vi "train_auto (deprecated).vi"() -> ()   [LabVIEW 2024]
uses:
  <vilib>/userDefined/High Color/IMAQdx.ctl
  <vilib>/vision/driver/NI_Vision_Acquisition_Software.lvlib
  <vilib>/vision/NI_Vision_Development_Module.lvlib
panel:
  in  "Set":enum16{"Train", "Test"}(ring)
  in  "Time Target (s)":dbl=0.4 min=0.1 max=20.0 step=0.1
  in  "Reset Set":bool
  in  "Update ROI":bool
  out "Original Image":T1(plugin-control)
  out "Time":dbl caption="Elapsed Time (s)"
  out "Toma":i32
  out "ROI":T1(plugin-control)
  in  "Save":bool
  in  "No. de Carta":i32
  in  "Path":string[](array[string])=["C:\\Users\\cesar\\OneDrive\\Universidad\\8vo Semestre\\Instrumentación Virtual 2\\Final\\cards\\train\\", "C:\\Users\\cesar\\OneDrive\\Universidad\\8vo Semestre\\Instrumentación Virtual 2\\Final\\cards\\test\\"]
  in  "Y":i32=150
  in  "X":i32=132
  out "Scaled ROI":T1(plugin-control)
  in  "ROI":T2={"Global Rectangle"=[408, 127, 510, 269], "Contours"=[{"Contour Type"=0, "ROI Type"=3, "Points"=[405, 125, 515, 272]}]}
  in  "Session In":T3="cam2"
  in  "Stop":bool
  # "Scale"
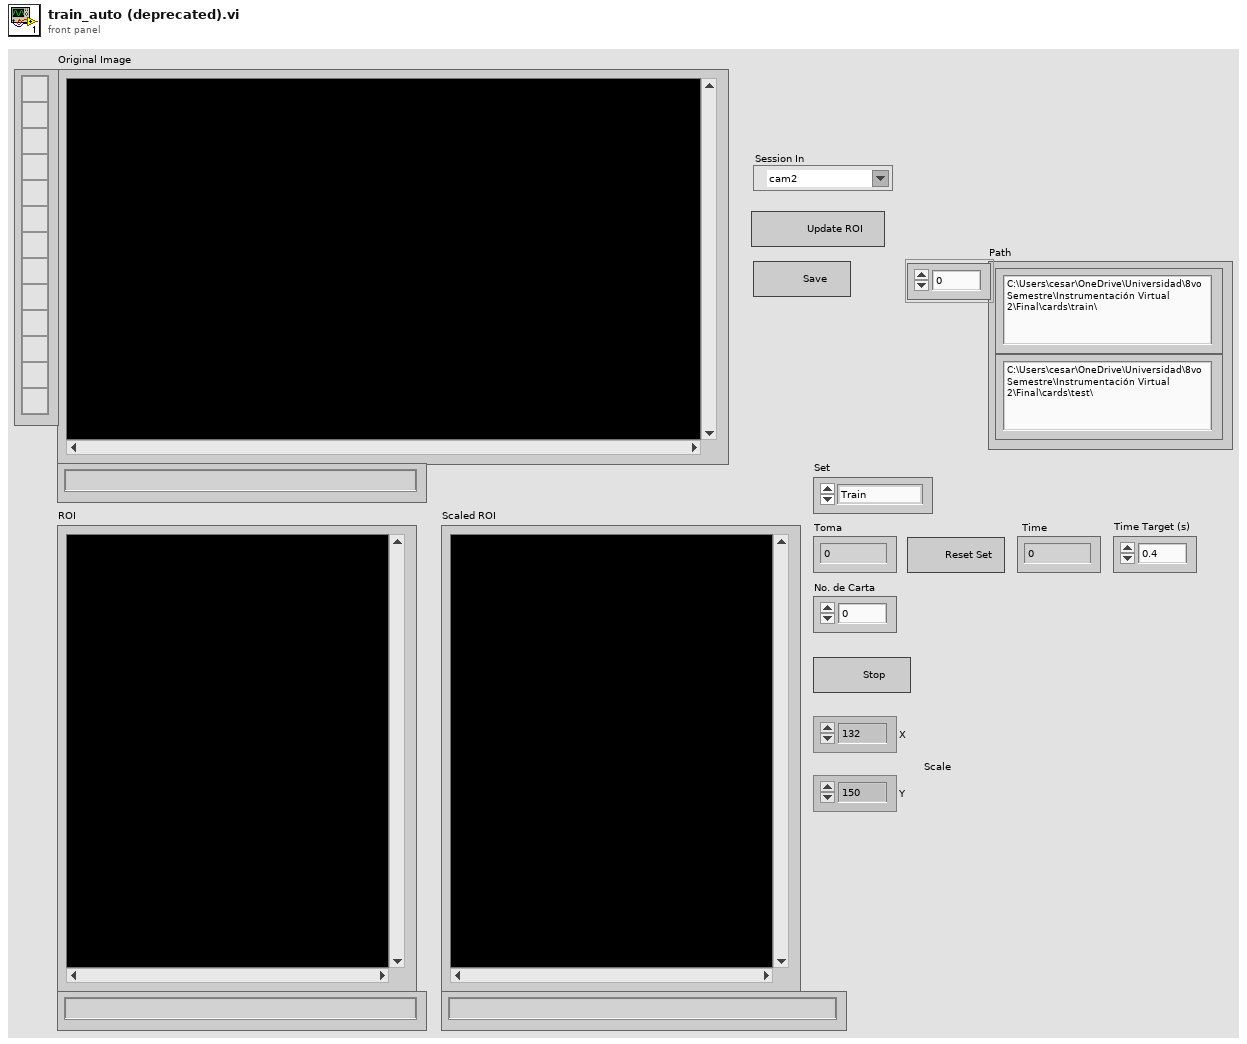
[diagram p1: front panel]
types:
  T1 = typedef "IMAQ Image.ctl" = refnum<image>
  T2 = cluster{"Global Rectangle":i32[], "Contours":cluster{"Contour Type":u32, "ROI Type":u32, "Points":i32[]}[]}
  T3 = typedef "IMAQdx.ctl" = refnum<k21>
  T4 = cluster{"Contour Type":u32, "ROI Type":u32, "Points":i32[]}[]
  T5 = cluster{"Contour Type":u32, "ROI Type":u32, "Points":i32[]}
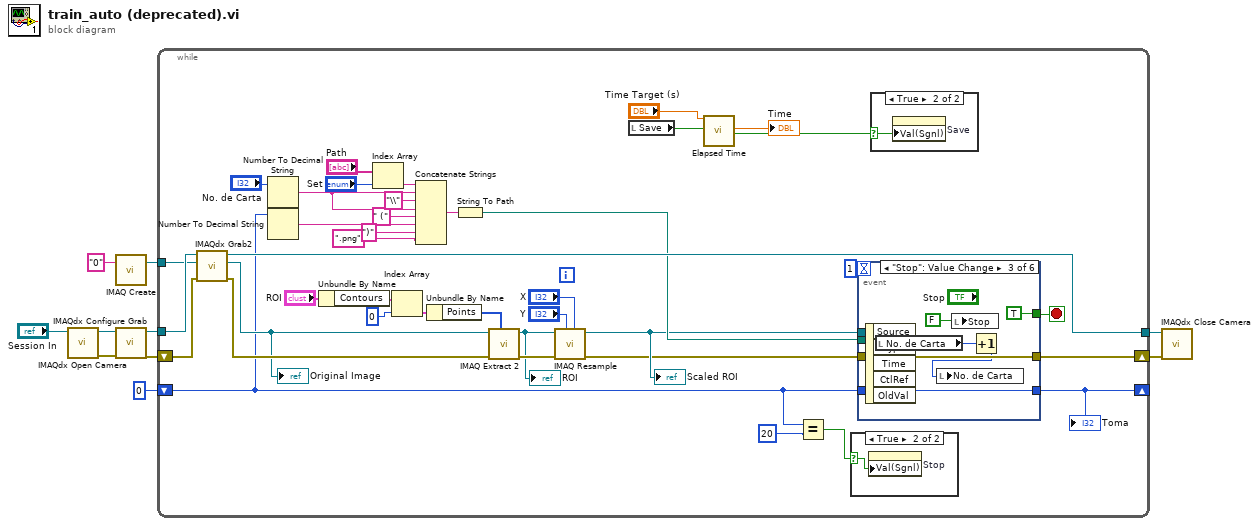
[diagram p0: block diagram]
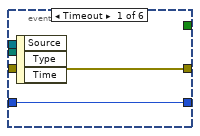
[diagram p4: hidden frame]
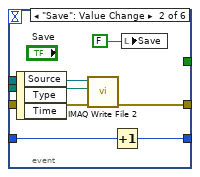
[diagram p5: hidden frame]
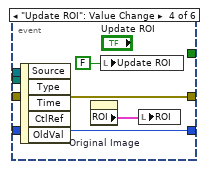
[diagram p6: hidden frame]
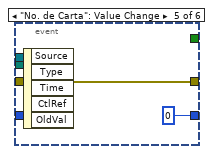
[diagram p7: hidden frame]
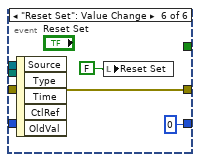
[diagram p8: hidden frame]
diagram:
  n1 = call <vilib>:"IMAQdx Open Camera.vi"("Session In"="Session In") -> ("error out"=w8:errorcluster, "Session Out"=w9:T3)  [unwired: 9 in]
  n2 = call "IMAQ Create"("Image Name"="0") -> ("New Image"=w5:T1)  [unwired: 4 in, 1 out]
  n3 = call <vilib>:"IMAQdx Configure Grab.vi"("error in"=w8, "Session In"=w9) -> ("error out"=w1:errorcluster, "Session Out"=w6:T3)  [unwired: 8 in]
  n4 = while {
    tunnel: w6 -> [w50]
    tunnel: w5 -> [w49]
    tunnel: [w48] -> w4
    shift-right: [w29] -> _
    shift-left: 0 -> [w14]
    shift-right: [w32] -> w3
    shift-left: w1 -> [w22]
    stop <- w12 stop-if-true
    n5 = call <vilib>:"IMAQdx Grab2.vi"("error in"=w22, "Image In"=w49, "Session In"=w50) -> ("error out"=w42:errorcluster, "Image Out"=w23:T1, "Session Out"=w48:T3)  [unwired: 5 in, 1 out]
    "Original Image" <- w23
    n6 = Number To Decimal String(number="No. de Carta") -> (decimal integer string=w38:string)  [unwired: 1 in]
    n7 = Number To Decimal String(number=w14) -> (decimal integer string=w36:string)  [unwired: 1 in]
    n8 = Unbundle By Name("ROI") -> ("Contours"=w47:T4)
    n9 = Index Array(array="Path", index="Set") -> (element=w18:string)
    n10 = Index Array(array=w47, index=0) -> (element=w45:T5)
    n11 = Concatenate Strings(w18, w38, "\\" ("string"), w38, " (" ("string"), w36, ")" ("string"), ".png" ("string")) -> (w17:string)
    n12 = Unbundle By Name(w45) -> ("Points"=w28:i32[])
    n13 = String To Path(string=w17) -> (path=w33:path)
    n14 = call "IMAQ Extract 2"("Optional Rectangle"=w28, "error in (no error)"=w42, "Image Src"=w23) -> ("error out"=w41:errorcluster, "Image Dst Out"=w27:T1)  [unwired: 7 in]
    "ROI" <- w27
    n15 = call "IMAQ Resample"("X Resolution"="X", "Y Resolution"="Y", "error in (no error)"=w41, "Image Src"=w27) -> ("error out"=w15:errorcluster, "Image Dst Out"=w16:T1)  [unwired: 6 in]
    "Scaled ROI" <- w16
    n16 = local read "Save"() -> (w25:bool)
    n17 = call "Elapsed Time"("Time Target (s)"="Time Target (s)", "Reset"=w25) -> ("Elapsed Time (s)"=→"Time":dbl, "Time has Elapsed"=w24:bool)  [unwired: 10 in, 6 out]
    n18 = Equal?(x=w14, y=20) -> (x = y?=w11:bool)
    n19 = case shown="True" w11 {
      selector: w11 -> [_ w51]
      frame False {
      }
      frame True {
        n20 = property on="Stop" class="Bool (strict)"("Val(Sgnl)"=w51) -> ()  [unwired: 2 in, 2 out]
      }
    }
    n21 = event shown="[2] \"Stop\": Value Change" {
      selector: _ -> [_ _ _ _ _ _]
      dyn-events: _ -> [_ _ _ _ _ _]
      timeout: 1 -> [_ _ _ _ _ _]
      tunnel: w15 -> [w54 w57 w66 w68 w73 w76]
      tunnel: w33 -> [_ w61 _ _ _ _]
      tunnel: w16 -> [_ w60 _ _ _ _]
      tunnel: [w54 w56 w66 w68 w73 w76] -> w32
      tunnel: w14 -> [w53 w59 w65 w69 _ _]
      tunnel: [w53 w58 w65 w69 0 0] -> w29
      tunnel: [_ _ TRUE _ _ _] -> w12
      event Timeout {
        n22 = event-data() -> ()  [unwired: 1 in, 3 out]
      }
      event "Save": Value Change {
        n23 = event-data() -> ()  [unwired: 1 in, 3 out]
        n24 = call-poly "IMAQ Write File 2"("error in (no error)"=w57, "File Path"=w61, "Image"=w60) -> ("error out"=w56:errorcluster)  [unwired: 7 in, 1 out]
        n25 = Increment(x=w59) -> (x+1=w58:i32)
        n26 = local write "Save"(FALSE ("Save")) -> ()
      }
      event "Stop": Value Change {
        n27 = event-data() -> ()  [unwired: 1 in, 5 out]
        n28 = local read "No. de Carta"() -> (w64:i32)
        n29 = local write "Stop"(FALSE) -> ()
        n30 = Increment(x=w64) -> (x+1=w63:i32)
        n31 = local write "No. de Carta"(w63) -> ()
      }
      event "Update ROI": Value Change {
        n32 = event-data() -> ()  [unwired: 1 in, 5 out]
        n33 = property on="Original Image" class="ImageControl"() -> ("ROI"=w70:T2)  [unwired: 2 in, 2 out]
        n34 = local write "Update ROI"(FALSE ("Update ROI")) -> ()
        n35 = local write "ROI"(w70) -> ()
      }
      event "No. de Carta": Value Change {
        n36 = event-data() -> ()  [unwired: 1 in, 5 out]
      }
      event "Reset Set": Value Change {
        n37 = event-data() -> ()  [unwired: 1 in, 5 out]
        n38 = local write "Reset Set"(FALSE ("Reset Set")) -> ()
      }
    }
    "Toma" <- w29
    n39 = case shown="True" w24 {
      selector: w24 -> [_ w52]
      frame False {
      }
      frame True {
        n40 = property on="Save" class="Bool (strict)"("Val(Sgnl)"=w52) -> ()  [unwired: 2 in, 2 out]
      }
    }
  }
  n41 = call <vilib>:"IMAQdx Close Camera.vi"("error in"=w3, "Session In"=w4) -> ()  [unwired: 9 in, 1 out]
